vi "run order display.vi"() -> ()   [LabVIEW 2016]
doc: "Displays Run Order for editting and monitoring"
uses:
  datarunorder.ctl
  <vilib>/Utility/miscctls.llb/LVRowAndColumnTypeDef.ctl
  <vilib>/addons/database/Connection.llb/DB Tools Open Connec (String).vi
  <vilib>/addons/database/Connection.llb/Conn Execute.vi
  <vilib>/addons/database/Recordset.llb/Rec Fetch Recordset Data (R).vi
  <vilib>/addons/database/Recordset.llb/Rec Destroy - Connection.vi
  <vilib>/addons/database/NI_Database_API.lvlib
panel:
  in  "Tab Control":enum32{"Main", "Arrays and data"}(tab)
  in  "stop":bool
  out "Time Remaining Property error":errorcluster
  out "Estimated Time Remaining(min)":sgl format="%#.1f"
  out "sequences remaining":u8(slide) scale=0.0..80.0
  in  "run order display":T1
  in  "edit run list":i32(listbox)
  in  "Total time for each sequence(min)":dbl
  out "Estimated Wheel Finish time and Date":timestamp format="%<%I:%M %p\n%x>T"
  out "Total number of sequence":i32
  out "Sequence remaining":i32
  out "Add Holder error":errorcluster
  out "empty?":bool
  in  "add holder":T2
  in  "update wheel numbers":bool
  out "position change":u32[][](array[colorbox])
  out "position":u32
  out "subarray 2":string[](array[string])
  in  "create wheel file":bool
  out "Add Holder error 2":errorcluster
  out "Array":i32[](array[numeric])
  out "Group run list":string[][](array[string])
  out "Data":T3(array[cluster])
  out "subarray":string[](array[string])
  out "outofrange":bool
  out "cathode data":string[](array[string])
  out "recordset data":variant[][](array[variant])
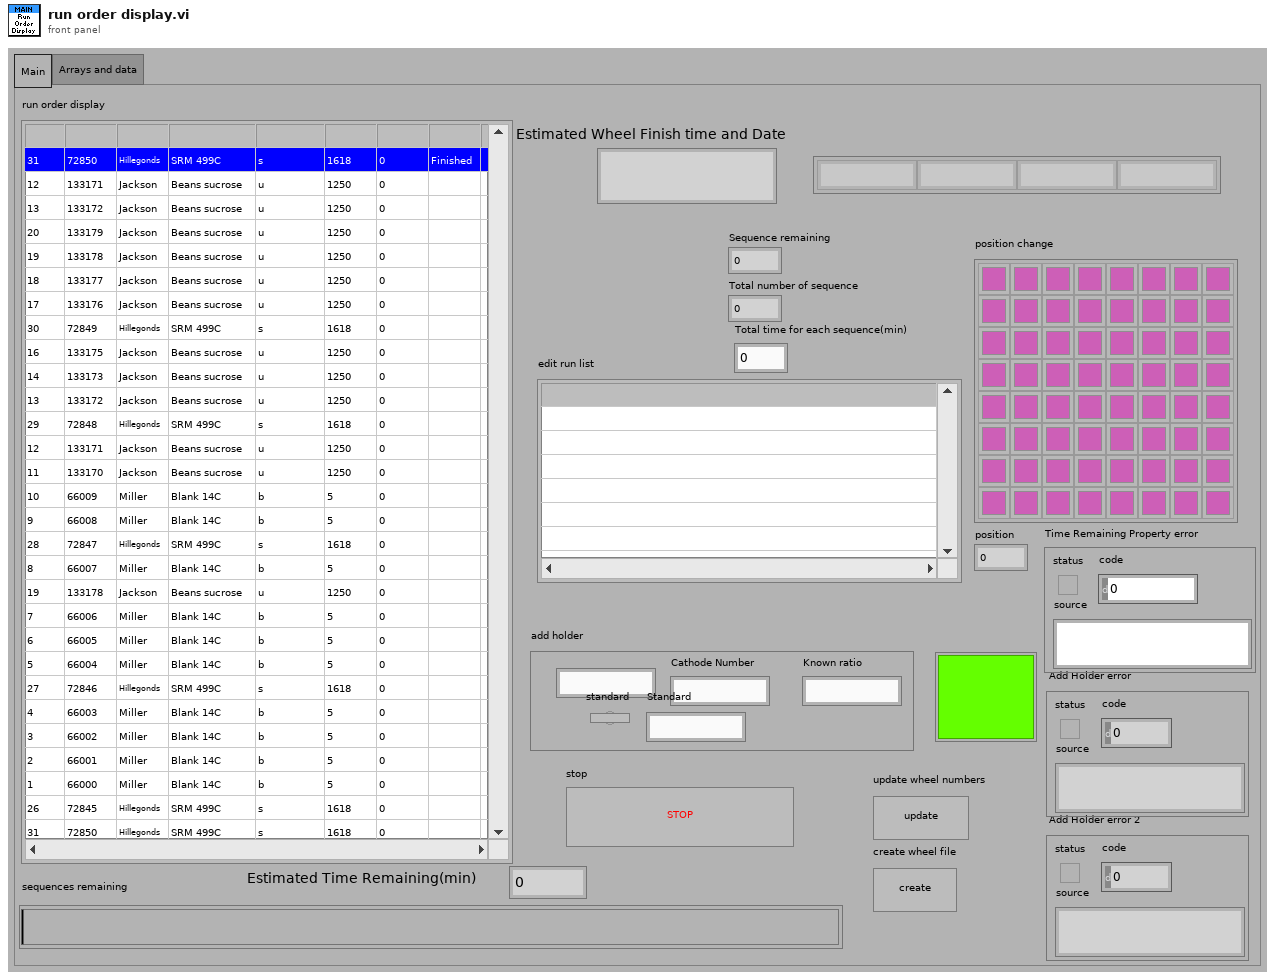
[diagram p1: front panel]
types:
  T1 = typedef "datarunorder.ctl" = i32
  T2 = cluster{"position":string, "Cathode Number":string, "standard":bool, "Known ratio":string, "Standard":string}
  T3 = cluster{"data name":string, "drag data":variant}[]
  T4 = typedef "LVRowAndColumnTypeDef.ctl" = cluster{"Row":i32, "Column":i32}
  T5 = typedef "LVPoint32TypeDef.ctl" = cluster{"Horizontal":i32, "Vertical":i32}
  T6 = typedef "NI_Database_API.lvlib/Conn ObjectReference.ctl" = refnum<k1>
  T7 = typedef "NI_Database_API.lvlib/Rec ObjectReference.ctl" = refnum<k1>
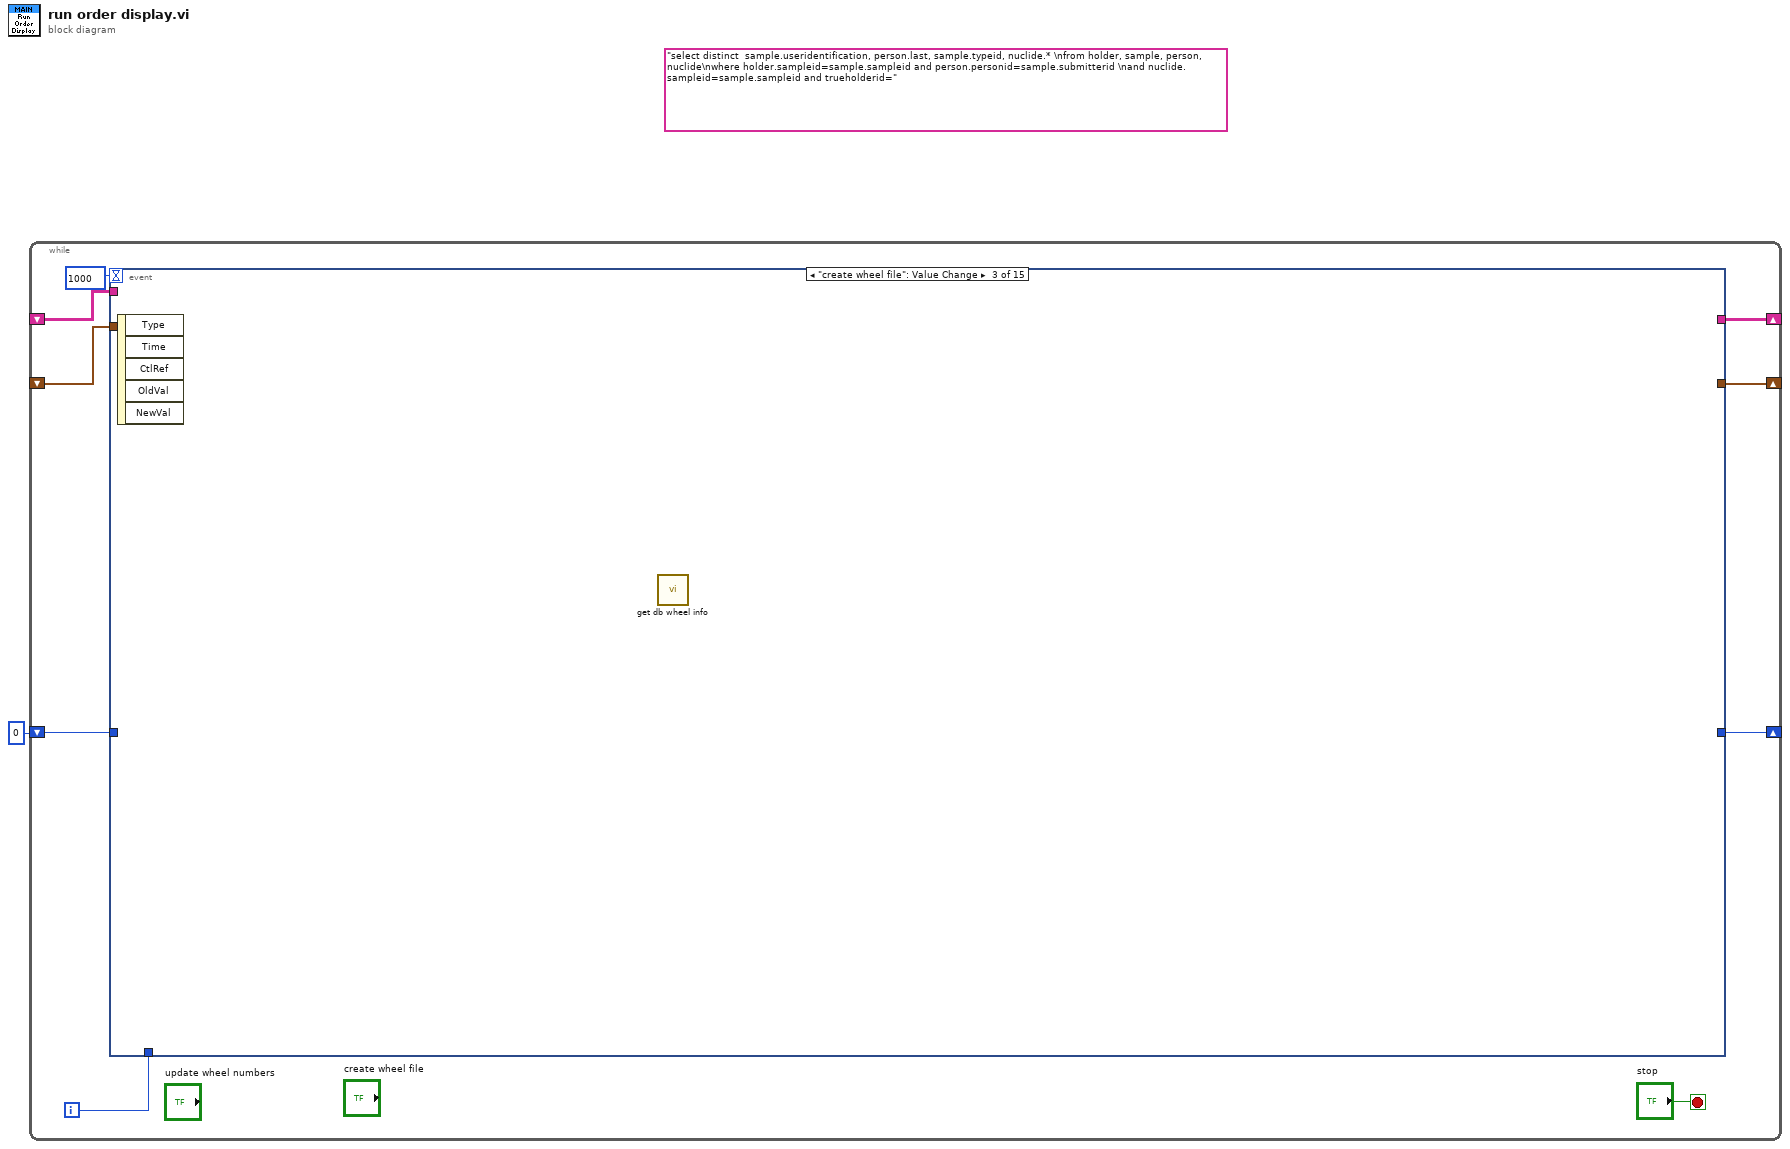
[diagram p0: block diagram]
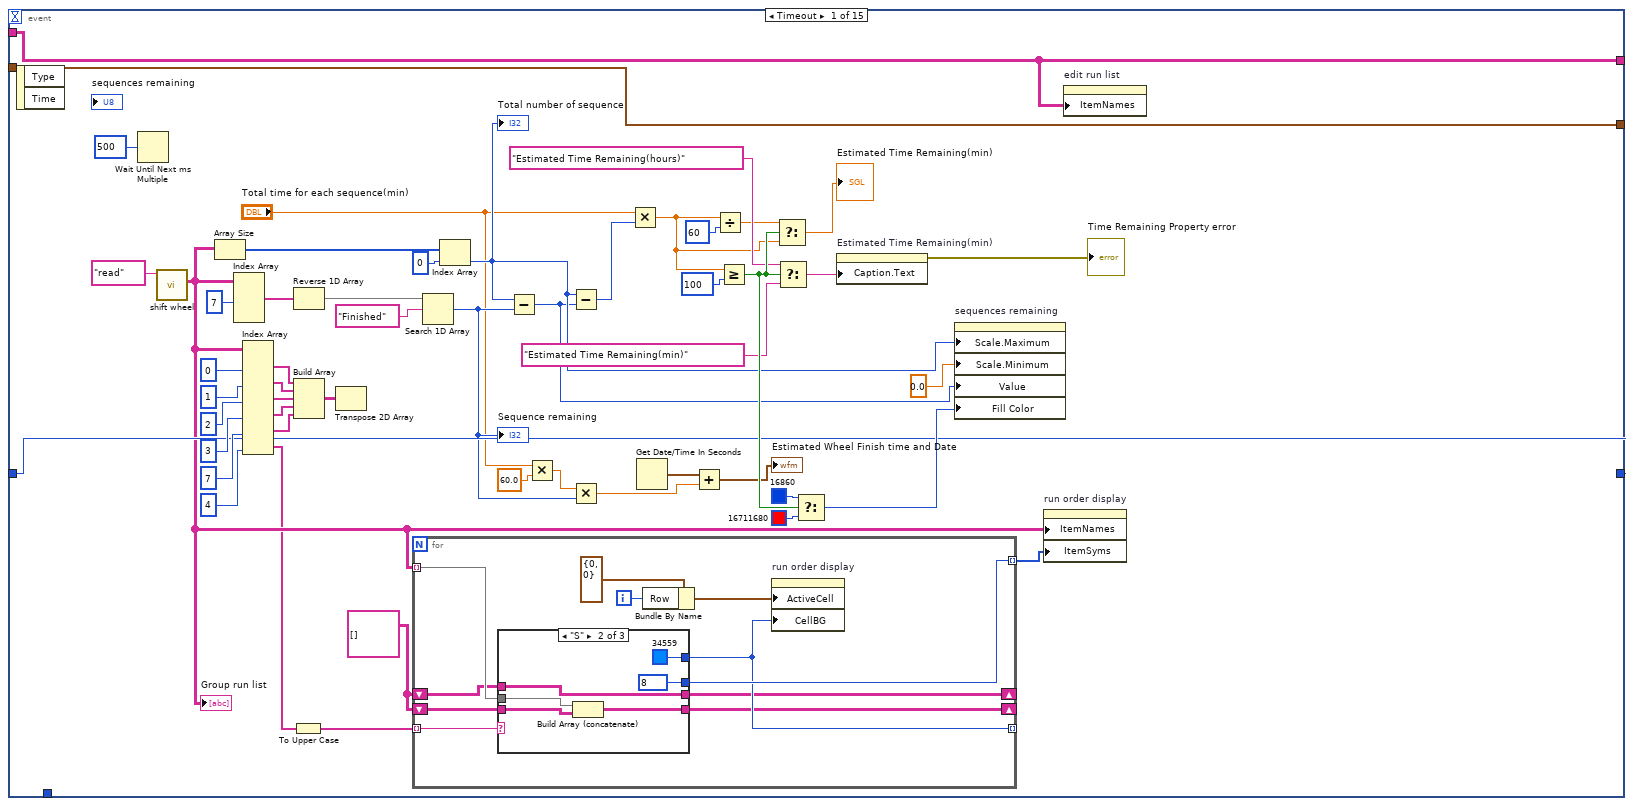
[diagram p2: hidden frame]
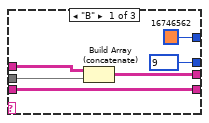
[diagram p3: hidden frame]
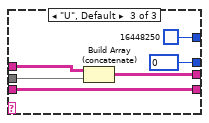
[diagram p4: hidden frame]
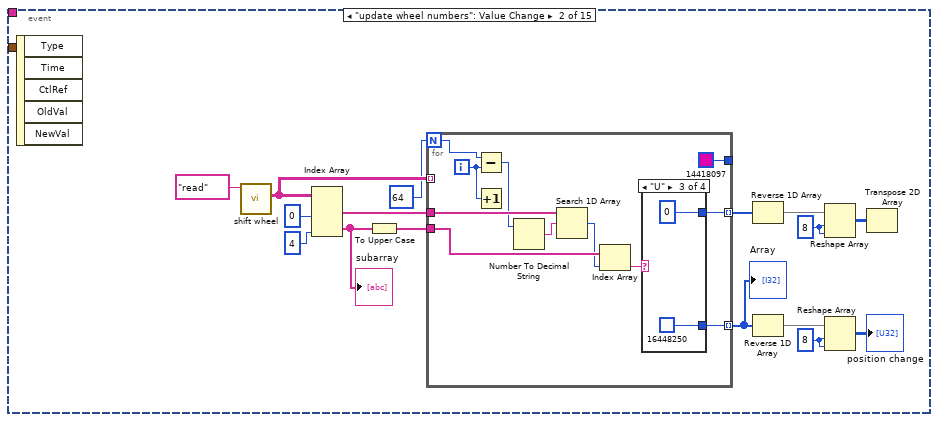
[diagram p5: hidden frame]
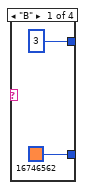
[diagram p6: hidden frame]
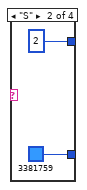
[diagram p7: hidden frame]
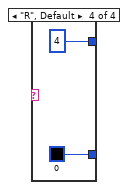
[diagram p8: hidden frame]
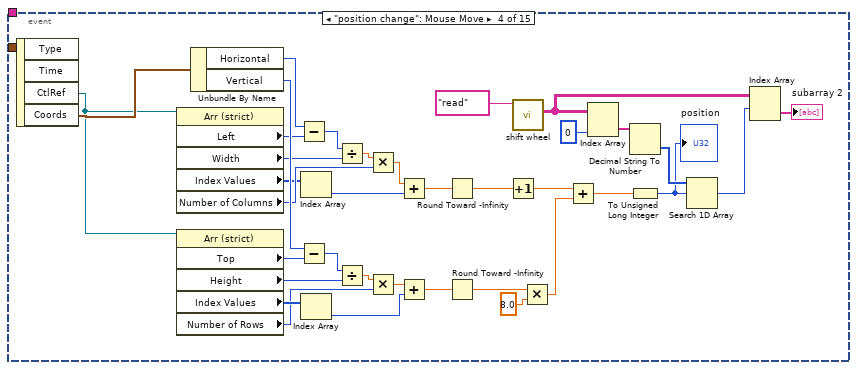
[diagram p9: hidden frame]
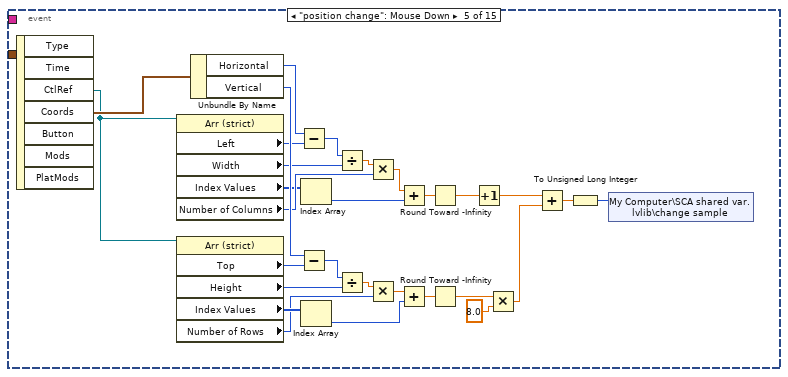
[diagram p10: hidden frame]
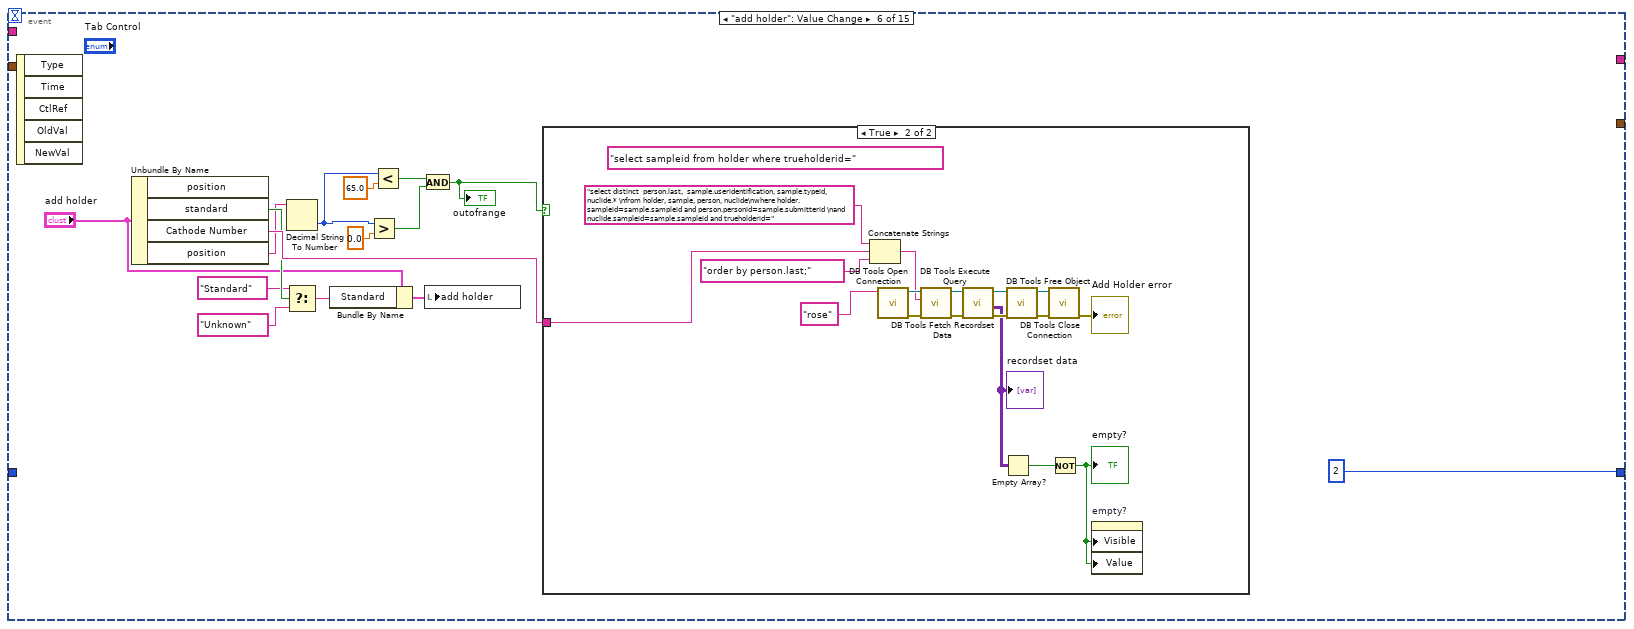
[diagram p11: hidden frame]
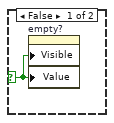
[diagram p12: hidden frame]
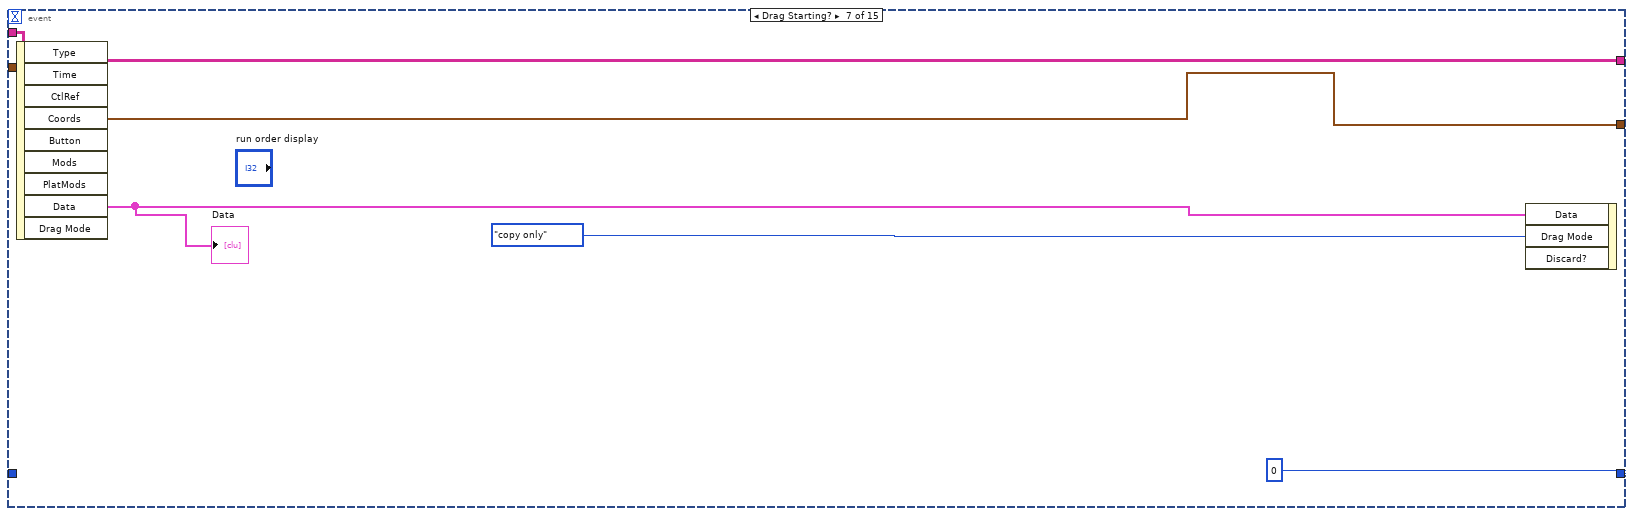
[diagram p13: hidden frame]
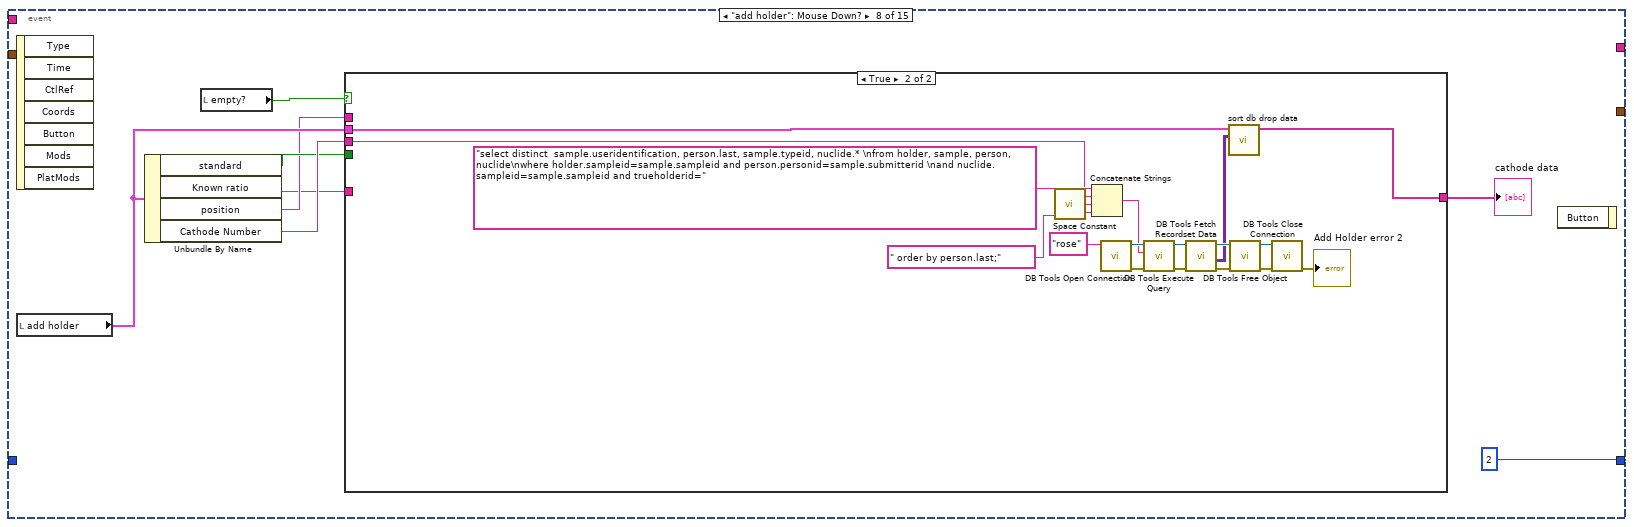
[diagram p14: hidden frame]
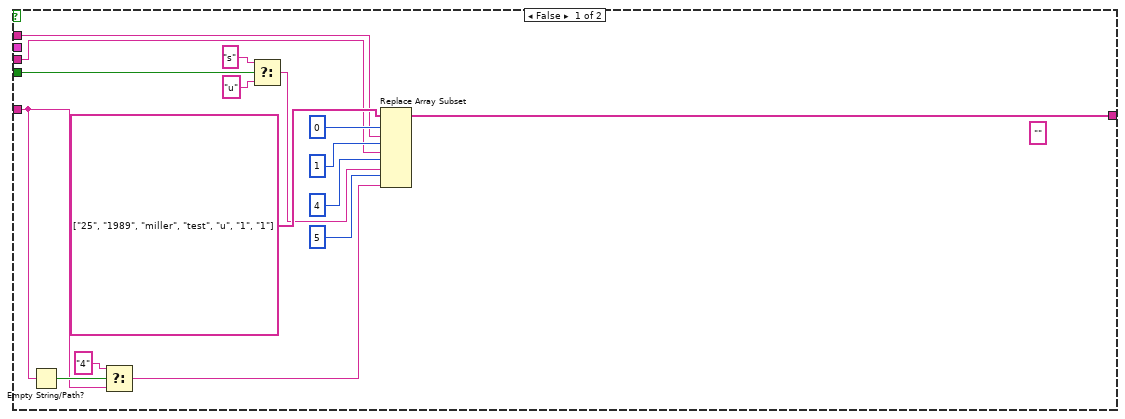
[diagram p15: hidden frame]
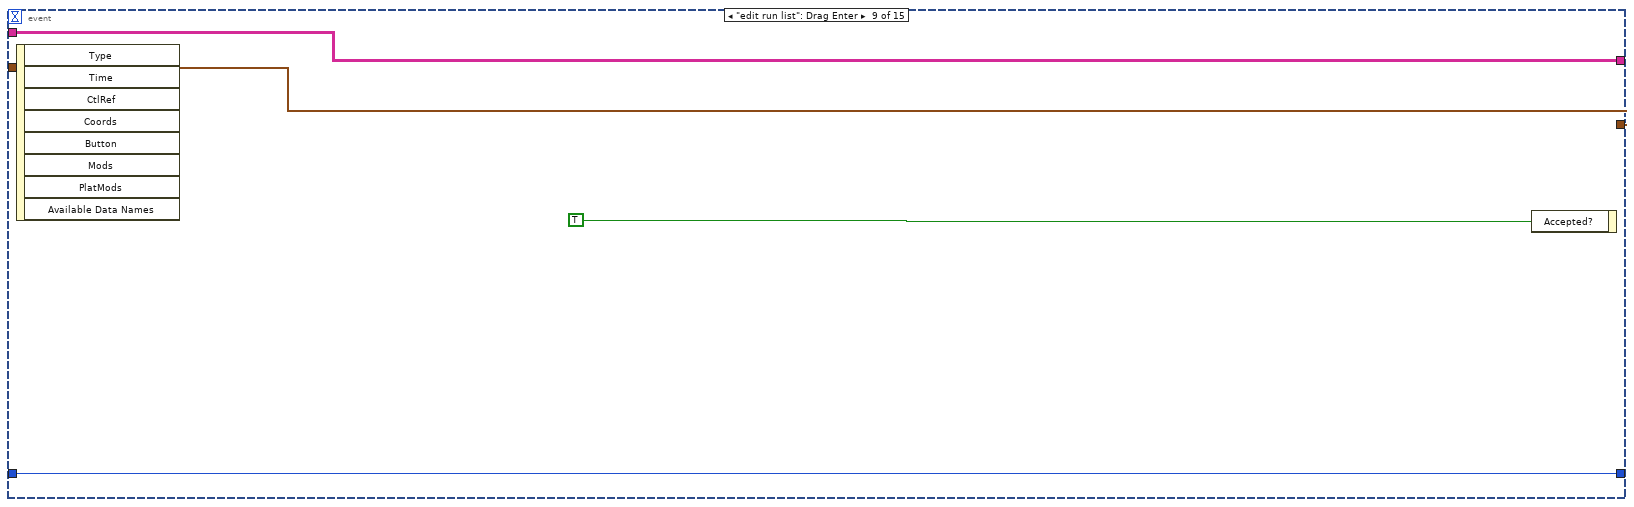
[diagram p16: hidden frame]
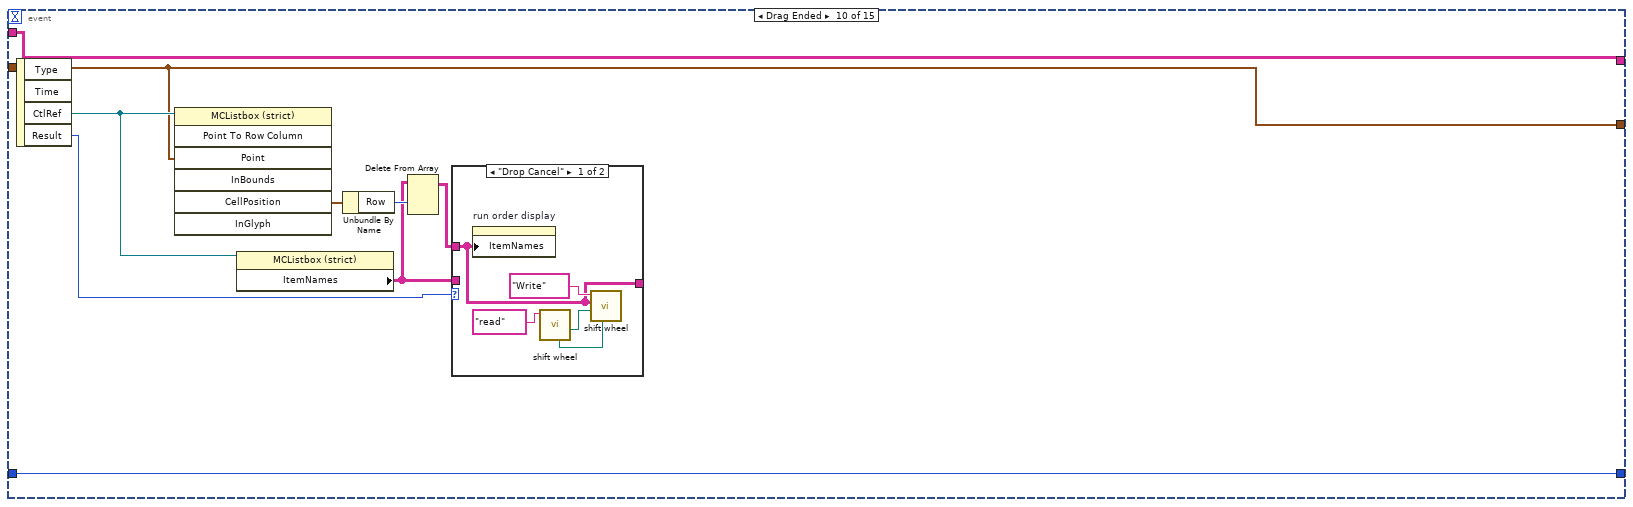
[diagram p17: hidden frame]
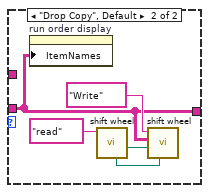
[diagram p18: hidden frame]
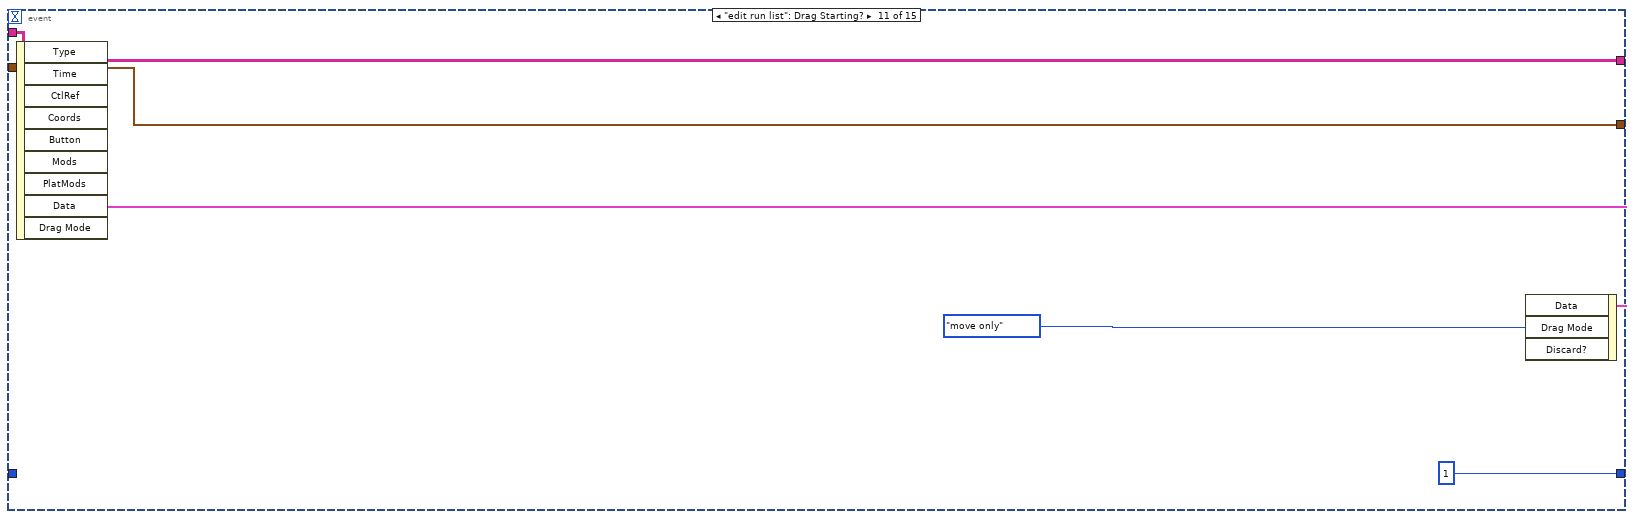
[diagram p19: hidden frame]
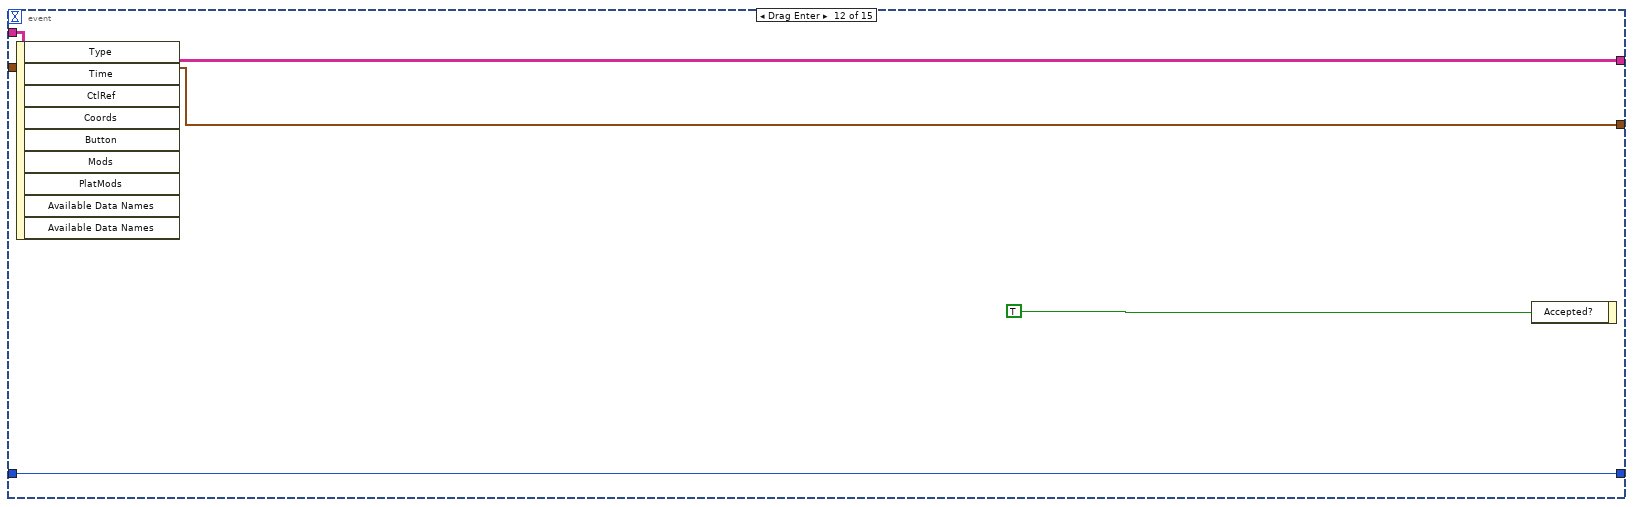
[diagram p20: hidden frame]
diagram:
  (unwired) "select distinct  sample.useridentification, person.last, sample.typeid, nuclide.* \nfrom holder, sample, person, nuclide\nwhere holder.sampleid=sample.sampleid and person.personid=sample.submitterid \nand nuclide.sampleid=sample.sampleid and trueholderid="
  n1 = while {
    shift-right: [w8] -> _
    shift-left: _ -> [w7]
    shift-right: [w6] -> _
    shift-left: _ -> [w5]
    shift-right: [w4] -> _
    shift-left: 0 -> [w3]
    i -> [w2]
    stop <- "stop" stop-if-true
    n2 = event shown="[2] \"create wheel file\": Value Change" {
      selector: _ -> [_ _ _ _ _ _ _ _ _ _ _ _ _ _ _]
      dyn-events: _ -> [_ _ _ _ _ _ _ _ _ _ _ _ _ _ _]
      timeout: 1000 -> [_ _ _ _ _ _ _ _ _ _ _ _ _ _ _]
      tunnel: w2 -> [_ _ _ _ _ _ _ _ _ _ _ _ _ _ _]
      tunnel: [w18 _ _ _ _ _ w228 _ w274 w277 w297 w302 _ _ w411] -> w8
      tunnel: w7 -> [w18 _ _ _ _ _ w228 _ w274 w277 w297 w302 w306 w356 w410]
      tunnel: [w62 _ _ _ _ _ w226 _ w273 w283 w296 w301 w315 w361 w406] -> w6
      tunnel: w5 -> [w62 _ _ _ _ _ _ _ w273 w283 w296 w301 w315 w361 w406]
      tunnel: [w26 _ _ _ _ 2 0 2 w272 w276 1 w300 0 0 w405] -> w4
      tunnel: w3 -> [w26 _ _ _ _ _ _ _ w272 w276 _ w300 w308 w359 w405]
      event Timeout {
        w15 = string[][] []
        n3 = event-data() -> ()  [unwired: 1 in, 2 out]
        n4 = Wait Until Next ms Multiple(millisecond multiple=u32 500) -> ()  [unwired: 1 out]
        n5 = call "shift wheel.vi"("read write"="read") -> ("Group run list"=w16:string[][])  [unwired: 8 in, 2 out]
        "Group run list" <- w16
        n6 = Array Size(array=w16) -> (size(s)=w28:i32[])
        n7 = Index Array(array=w16, index (col) #1=7 ("disabled index (col)")) -> (element #1=w31:string[])  [unwired: 3 in, 1 out]
        n8 = Index Array(array=w16, index (col) #1=0 ("disabled index (col)"), index (col) #2=1 ("index (col)"), index (col) #3=2 ("index (col)"), index (col) #4=3 ("index (col)"), index (col) #5=7 ("index (col)"), index (col) #6=4 ("index (col)")) -> (element #1=w56:string[], element #2=w57:string[], element #3=w58:string[], element #4=w59:string[], element #5=w60:string[], element #6=w13:string[])  [unwired: 6 in]
        n9 = To Upper Case(1:w13) -> (0:w12:string[])
        n10 = Reverse 1D Array(array=w31) -> (reversed array=w32:string[])
        n11 = Build Array(w56, w57, w58, w59, w60) -> (w61:string[][])
        n12 = Transpose 2D Array(2D array=w61) -> ()  [unwired: 1 out]
        n13 = for {
          tunnel: w12 -> [w73] mode=indexing
          tunnel: [w72] -> w14 mode=indexing
          tunnel: [w69] -> _ mode=indexing
          tunnel: w16 -> [w67] mode=indexing
          shift-right: [w66] -> _
          shift-left: w15 -> [w65]
          shift-right: [w64] -> _
          shift-left: w15 -> [w63]
          i -> [w68]
          n14 = case shown="\"S\"" w73 {
            tunnel: [9 8 0] -> w72
            tunnel: [u32 16746562 u32 34559 u32 16448250] -> w69
            tunnel: w67 -> [w74 w82 w88]
            tunnel: [w77 w83 w87] -> w66
            tunnel: w65 -> [w75 w83 w89]
            tunnel: [w76 w81 w86] -> w64
            tunnel: w63 -> [w76 w80 w86]
            frame "B" {
              n15 = Build Array (concatenate)(w75, w74) -> (w77:string[][])
            }
            frame "S" {
              n16 = Build Array (concatenate)(w82, w80) -> (w81:string[][])
            }
            frame "U", Default {
              n17 = Build Array (concatenate)(w89, w88) -> (w87:string[][])
            }
          }
          n18 = Bundle By Name(cluster=T4 {"Row"=0, "Column"=0} ("Active Cell:Active Cell"), "Row"=w68) -> (w71:T4)
          n19 = property on="run order display" class="MCListbox (strict)"("ActiveCell"=w71, "CellBG"=w69) -> ()  [unwired: 2 in, 2 out]
        }
        n20 = Search 1D Array(1D array=w32, element="Finished") -> (index of element=w20:i32)  [unwired: 1 in]
        "Sequence remaining" <- w20
        n21 = Index Array(array=w28, index=0) -> (element=w36:i32)
        "Total number of sequence" <- w36
        n22 = Subtract(x=w36, y=w20) -> (x-y=w24:i32)
        n23 = Multiply(x="Total time for each sequence(min)", y=60.0) -> (x*y=w22:dbl)
        n24 = Subtract(x=w36, y=w24) -> (x-y=w37:i32)
        n25 = Multiply(x=w22, y=w20) -> (x*y=w21:dbl)
        n26 = Multiply(x="Total time for each sequence(min)", y=w37) -> (x*y=w39:dbl)
        n27 = Get Date/Time In Seconds() -> (seconds since 1Jan1904=w25:timestamp)
        n28 = Add(x=w25, y=w21) -> (x+y=→"Estimated Wheel Finish time and Date":timestamp)
        n29 = Divide(x=w39, y=60) -> (x/y=w41:dbl)
        n30 = Greater Or Equal?(x=w39, y=100) -> (x >= y?=w49:bool)
        n31 = Select(t=w41, s=w49, f=w39) -> (s? t:f=→"Estimated Time Remaining(min)":dbl)
        n32 = Select(t="Estimated Time Remaining(hours)" ("Label.Text"), s=w49, f="Estimated Time Remaining(min)" ("Label.Text")) -> (s? t:f=w46:string)
        n33 = Select(t=u32 16860 ("Color Box"), s=w49, f=u32 16711680 ("Color Box 2")) -> (s? t:f=w50:u32)
        n34 = property on="Estimated Time Remaining(min)" class="DigNum (strict)"("Caption.Text"=w46) -> (error out=→"Time Remaining Property error":errorcluster)  [unwired: 2 in, 1 out]
        n35 = property on="sequences remaining" class="Slide (strict)"("Scale.Maximum"=w36, "Scale.Minimum"=0.0 ("Scale.Range:Minimum"), "Value"=w24, "Fill Color"=w50) -> ()  [unwired: 2 in, 2 out]
        n36 = property on="run order display" class="MCListbox (strict)"("ItemNames"=w16, "ItemSyms"=w14) -> ()  [unwired: 2 in, 2 out]
        n37 = property on="edit run list" class="MCListbox (strict)"("ItemNames"=w18) -> ()  [unwired: 2 in, 2 out]
      }
      event "update wheel numbers": Value Change {
        w96 = 8 ("dimension size")
        w99 = 8 ("dimension size")
        n38 = event-data() -> ()  [unwired: 1 in, 5 out]
        n39 = call "shift wheel.vi"("read write"="read") -> ("Group run list"=w106:string[][])  [unwired: 8 in, 2 out]
        n40 = Index Array(array=w106, index (col) #1=0 ("disabled index (col)"), index (col) #2=4 ("index (col)")) -> (element #1=w103:string[], element #2=w101:string[])  [unwired: 2 in]
        "subarray" <- w101
        n41 = To Upper Case(1:w101) -> (0:w100:string[])
        n42 = for {
          N: 64 -> [w112]
          tunnel: w106 -> [_] mode=indexing
          tunnel: w103 -> [w118]
          tunnel: w100 -> [w116]
          tunnel: [w113] -> w98 mode=indexing
          tunnel: [u32 14418097 ("Color Box")] -> _
          tunnel: [w108] -> w95 mode=indexing
          i -> [w111]
          n43 = Subtract(x=w112, y=w111) -> (x-y=w110:i32)
          n44 = Increment(x=w111) -> ()  [unwired: 1 out]
          n45 = Number To Decimal String(number=w110) -> (decimal integer string=w117:string)  [unwired: 1 in]
          n46 = Search 1D Array(1D array=w118, element=w117) -> (index of element=w115:i32)  [unwired: 1 in]
          n47 = Index Array(array=w116, index=w115) -> (element=w114:string)
          n48 = case shown="\"U\"" w114 {
            tunnel: [u32 16746562 ("Color Box") u32 3381759 ("Color Box") u32 16448250 ("Color Box") u32 0 ("Color Box")] -> w113
            tunnel: [3 ("x") 2 ("x") 0 ("x") 4 ("x")] -> w108
            frame "B" {
            }
            frame "S" {
            }
            frame "U" {
            }
            frame "R", Default {
            }
          }
        }
        "Array" <- w98
        n49 = Reverse 1D Array(array=w95) -> (reversed array=w94:i32[])
        n50 = Reverse 1D Array(array=w98) -> (reversed array=w97:u32[])
        n51 = Reshape Array(w94, w96, w96) -> (w93:i32[][])
        n52 = Reshape Array(w97, w99, w99) -> (→"position change":u32[][])
        n53 = Transpose 2D Array(2D array=w93) -> ()  [unwired: 1 out]
      }
      event "create wheel file": Value Change {
        n54 = event-data() -> ()  [unwired: 1 in, 5 out]
        n55 = call "get db wheel info.vi"() -> ()  [unwired: 1 in]
      }
      event "position change": Mouse Move {
        n56 = event-data() -> ("CtlRef"=w151:refnum<vi>, "Coords"=w161:T5)  [unwired: 1 in, 2 out]
        n57 = property class="Arr (strict)"(reference=w151) -> ("Left"=w145:i32, "Width"=w143:u32, "Index Values"=w141:u32[], "Number of Columns"=w142:u32)  [unwired: 1 in, 2 out]
        n58 = property class="Arr (strict)"(reference=w151) -> ("Top"=w159:i32, "Height"=w157:u32, "Index Values"=w156:u32[], "Number of Rows"=w155:u32)  [unwired: 1 in, 2 out]
        n59 = Unbundle By Name(w161) -> ("Horizontal"=w144:i32, "Vertical"=w160:i32)
        n60 = Subtract(x=w144, y=w145) -> (x-y=w147:i32)
        n61 = Subtract(x=w160, y=w159) -> (x-y=w158:i32)
        n62 = Index Array(array=w141) -> (element=w149:u32)  [unwired: 1 in]
        n63 = Index Array(array=w156) -> (element=w153:u32)  [unwired: 1 in]
        n64 = Divide(x=w147, y=w143) -> (x/y=w148:dbl)
        n65 = Divide(x=w158, y=w157) -> (x/y=w154:dbl)
        n66 = Multiply(x=w148, y=w142) -> (x*y=w150:dbl)
        n67 = Multiply(x=w154, y=w155) -> (x*y=w152:dbl)
        n68 = Add(x=w150, y=w149) -> (x+y=w146:dbl)
        n69 = Add(x=w152, y=w153) -> (x+y=w162:dbl)
        n70 = Round Toward -Infinity(1:w146) -> (0:w137:dbl)
        n71 = Round Toward -Infinity(1:w162) -> (0:w140:dbl)
        n72 = Increment(x=w137) -> (x+1=w136:dbl)
        n73 = call "shift wheel.vi"("read write"="read") -> ("Group run list"=w130:string[][])  [unwired: 8 in, 2 out]
        n74 = Multiply(x=w140, y=8.0) -> (x*y=w138:dbl)
        n75 = Add(x=w136, y=w138) -> (x+y=w133:dbl)
        n76 = Index Array(array=w130, index (col)=0 ("disabled index (col)")) -> (element=w134:string[])  [unwired: 1 in]
        n77 = Decimal String To Number(string=w134) -> (number=w132:i32[])  [unwired: 2 in, 1 out]
        n78 = To Unsigned Long Integer(number=w133) -> (unsigned 32bit integer=w131:u32)
        "position" <- w131
        n79 = Search 1D Array(1D array=w132, element=w131) -> (index of element=w129:i32)  [unwired: 1 in]
        n80 = Index Array(array=w130, index (row)=w129) -> (element=→"subarray 2":string[])  [unwired: 1 in]
      }
      event "position change": Mouse Down {
        n81 = event-data() -> ("CtlRef"=w180:refnum<vi>, "Coords"=w190:T5)  [unwired: 1 in, 5 out]
        n82 = property class="Arr (strict)"(reference=w180) -> ("Left"=w174:i32, "Width"=w172:u32, "Index Values"=w170:u32[], "Number of Columns"=w171:u32)  [unwired: 1 in, 2 out]
        n83 = property class="Arr (strict)"(reference=w180) -> ("Top"=w188:i32, "Height"=w186:u32, "Index Values"=w185:u32[], "Number of Rows"=w184:u32)  [unwired: 1 in, 2 out]
        n84 = Unbundle By Name(w190) -> ("Horizontal"=w173:i32, "Vertical"=w189:i32)
        n85 = Subtract(x=w173, y=w174) -> (x-y=w176:i32)
        n86 = Subtract(x=w189, y=w188) -> (x-y=w187:i32)
        n87 = Index Array(array=w170) -> (element=w178:u32)  [unwired: 1 in]
        n88 = Index Array(array=w185) -> (element=w182:u32)  [unwired: 1 in]
        n89 = Divide(x=w176, y=w172) -> (x/y=w177:dbl)
        n90 = Divide(x=w187, y=w186) -> (x/y=w183:dbl)
        n91 = Multiply(x=w177, y=w171) -> (x*y=w179:dbl)
        n92 = Multiply(x=w183, y=w184) -> (x*y=w181:dbl)
        n93 = Add(x=w179, y=w178) -> (x+y=w175:dbl)
        n94 = Add(x=w181, y=w182) -> (x+y=w191:dbl)
        n95 = Round Toward -Infinity(1:w175) -> (0:w166:dbl)
        n96 = Round Toward -Infinity(1:w191) -> (0:w169:dbl)
        n97 = Increment(x=w166) -> (x+1=w165:dbl)
        n98 = Multiply(x=w169, y=8.0) -> (x*y=w167:dbl)
        n99 = Add(x=w165, y=w167) -> (x+y=w164:dbl)
        n100 = To Unsigned Long Integer(number=w164) -> (unsigned 32bit integer=w163:u32)
        n101 = shared-variable "My Computer\\SCA shared var.lvlib\\change sample"(w163) -> ()  [unwired: 1 in, 1 out]
      }
      event "add holder": Value Change {
        n102 = event-data() -> ()  [unwired: 1 in, 5 out]
        n103 = Unbundle By Name("add holder") -> ("standard"=w202:bool, "Cathode Number"=w203:string, "position"=w196:string)  [unwired: 1 out]
        n104 = Decimal String To Number(string=w196) -> (number=w195:i32)  [unwired: 2 in, 1 out]
        n105 = Select(t="Standard" ("decimal integer string"), s=w202, f="Unknown" ("decimal integer string")) -> (s? t:f=w199:string)
        n106 = Bundle By Name(cluster="add holder", "Standard"=w199) -> (w198:T2)
        n107 = Greater?(x=w195, y=0.0) -> (0:w206:bool)
        n108 = Less?(x=w195, y=65.0) -> (x < y?=w205:bool)
        n109 = And(x=w205, y=w206) -> (x .and. y?=w204:bool)
        "outofrange" <- w204
        n110 = local write "add holder"(w198) -> ()
        n111 = case shown="True" w204 {
          selector: w204 -> [w207 _]
          tunnel: w203 -> [_ w211]
          frame False {
            n112 = property on="empty?" class="Bool (strict)"("Visible"=w207, "Value"=w207) -> ()  [unwired: 2 in, 2 out]
          }
          frame True {
            (unwired) "select sampleid from holder where trueholderid=" ("SQL query")
            n113 = Concatenate Strings("select distinct  person.last,  sample.useridentification, sample.typeid, nuclide.* \nfrom holder, sample, person, nuclide\nwhere holder.sampleid=sample.sampleid and person.personid=sample.submitterid \nand nuclide.sampleid=sample.sampleid and trueholderid=", w211, "order by person.last;" ("string")) -> (w219:string)
            n114 = call-poly <vilib>:"DB Tools Open Connection.vi"("connection information"="rose" ("decimal integer string")) -> ("error out"=w224:errorcluster, "connection reference"=w223:T6)  [unwired: 7 in]
            n115 = call-poly <vilib>:"DB Tools Execute Query.vi"("error in (no error)"=w224, "SQL query"=w219, "connection reference"=w223) -> ("error out"=w222:errorcluster, "recordset reference"=w221:T7)  [unwired: 5 in]
            n116 = call-poly <vilib>:"DB Tools Fetch Recordset Data.vi"("error in (no error)"=w222, "recordset reference"=w221) -> ("error out"=w218:errorcluster, "recordset data"=w213:variant[][], "recordset reference out"=w217:T7)  [unwired: 3 in]
            "recordset data" <- w213
            n117 = Empty Array?(array=w213) -> (empty?=w209:bool)
            n118 = call-poly <vilib>:"DB Tools Free Object.vi"("error in (no error)"=w218, "recordset reference"=w217) -> ("error out"=w216:errorcluster, "connection reference"=w215:T6)  [unwired: 8 in]
            n119 = call <vilib>:"DB Tools Close Connection.vi"("error in (no error)"=w216, "connection reference"=w215) -> ("error out"=→"Add Holder error":errorcluster)  [unwired: 5 in]
            n120 = Not(x=w209) -> (.not. x?=w208:bool)
            "empty?" <- w208
            n121 = property on="empty?" class="Bool (strict)"("Visible"=w208, "Value"=w208) -> ()  [unwired: 2 in, 2 out]
          }
        }
      }
      event Drag Starting? {
        n122 = event-data() -> ("Coords"=w226:T5, "Data"=w229:T3)  [unwired: 1 in, 7 out]
        "Data" <- w229
        n123 = event-data("Data"=w229, "Drag Mode"=enum32{"copy or move", "copy only", "move only"}."copy only") -> ()  [unwired: 2 in, 1 out]
      }
      event "add holder": Mouse Down? {
        n124 = event-data() -> ()  [unwired: 1 in, 7 out]
        n125 = local read "add holder"() -> (w235:T2)
        n126 = Unbundle By Name(w235) -> ("standard"=w233:bool, "Known ratio"=w231:string, "position"=w232:string, "Cathode Number"=w236:string)
        n127 = local read "empty?"() -> (w237:bool)
        n128 = case shown="True" w237 {
          tunnel: w236 -> [w246 w259]
          tunnel: w235 -> [_ w255]
          tunnel: [w238 w254] -> w230
          tunnel: w233 -> [w252 _]
          tunnel: w232 -> [w247 _]
          tunnel: w231 -> [w241 _]
          frame False {
            (unwired) "" ("new element/subarray")
            n129 = Empty String/Path?(string/path=w241) -> (empty?=w242:bool)
            n130 = Select(t="4" ("new element/subarray"), s=w242, f=w241) -> (s? t:f=w239:string)
            n131 = Select(t="s", s=w252, f="u") -> (s? t:f=w244:string)
            n132 = Replace Array Subset(array=string[] ["25", "1989", "miller", "test", "u", "1", "1"] ("cathode data"), new element #1=w247, index #1=0 ("index"), new element #2=w246, index #2=1 ("index"), new element #3=w244, index #3=4 ("index"), new element #4=w239, index #4=5 ("index")) -> (w238:string[])
          }
          frame True {
            n133 = call <vilib>:"Space Constant.vi"() -> ("String"=w257:string)
            n134 = Concatenate Strings("select distinct  sample.useridentification, person.last, sample.typeid, nuclide.* \nfrom holder, sample, person, nuclide\nwhere holder.sampleid=sample.sampleid and person.personid=sample.submitterid \nand nuclide.sampleid=sample.sampleid and trueholderid=", w259, w257, " order by person.last;" ("string")) -> (w263:string)
            n135 = call-poly <vilib>:"DB Tools Open Connection.vi"("connection information"="rose" ("decimal integer string")) -> ("error out"=w270:errorcluster, "connection reference"=w269:T6)  [unwired: 7 in]
            n136 = call-poly <vilib>:"DB Tools Execute Query.vi"("error in (no error)"=w270, "SQL query"=w263, "connection reference"=w269) -> ("error out"=w268:errorcluster, "recordset reference"=w267:T7)  [unwired: 5 in]
            n137 = call-poly <vilib>:"DB Tools Fetch Recordset Data.vi"("error in (no error)"=w268, "recordset reference"=w267) -> ("error out"=w262:errorcluster, "recordset data"=w256:variant[][], "recordset reference out"=w266:T7)  [unwired: 3 in]
            n138 = call "sort db drop data.vi"("recordset data"=w256, "add holder"=w255) -> ("cathode data"=w254:string[])  [unwired: 8 in, 1 out]
            n139 = call-poly <vilib>:"DB Tools Free Object.vi"("error in (no error)"=w262, "recordset reference"=w266) -> ("error out"=w261:errorcluster, "connection reference"=w265:T6)  [unwired: 8 in]
            n140 = call <vilib>:"DB Tools Close Connection.vi"("error in (no error)"=w261, "connection reference"=w265) -> ("error out"=→"Add Holder error 2":errorcluster)  [unwired: 5 in]
          }
        }
        "cathode data" <- w230
        n141 = event-data() -> ()  [unwired: 2 in, 1 out]
      }
      event "edit run list": Drag Enter {
        n142 = event-data() -> ()  [unwired: 1 in, 8 out]
        n143 = event-data("Accepted?"=TRUE) -> ()  [unwired: 1 in, 1 out]
      }
      event Drag Ended {
        n144 = event-data() -> ("CtlRef"=w284:refnum<vi>, "Result"=w279:enum16{"Drop Cancel", "Drop Move", "Drop Copy"})  [unwired: 1 in, 2 out]
        n145 = invoke class="MCListbox (strict)" method="Point To Row Column"(reference=w284, "Point"=w283) -> ("CellPosition"=w282:T4)  [unwired: 5 in, 6 out]
        n146 = property class="MCListbox (strict)"(reference=w284) -> ("ItemNames"=w278:string[][])  [unwired: 1 in, 2 out]
        n147 = Unbundle By Name(w282) -> ("Row"=w281:i32)
        n148 = Delete From Array(array=w278, index (row)=w281) -> (array with subset deleted=w280:string[][])  [unwired: 2 in, 1 out]
        n149 = case shown="\"Drop Cancel\"" w279 {
          tunnel: w280 -> [w285 _]
          tunnel: [w285 w290] -> _
          tunnel: w278 -> [_ w290]
          frame "Drop Cancel" {
            n150 = property on="run order display" class="MCListbox (strict)"("ItemNames"=w285) -> ()  [unwired: 2 in, 2 out]
            n151 = call "shift wheel.vi"("read write"="read") -> ("cycle results name out"=w288:path, "seq results name out"=w289:path)  [unwired: 8 in, 1 out]
            n152 = call "shift wheel.vi"("seq results name in"=w289, "cycle results name in"=w288, "Group run list write"=w285, "read write"="Write") -> ()  [unwired: 5 in, 3 out]
          }
          frame "Drop Copy", Default {
            n153 = property on="run order display" class="MCListbox (strict)"("ItemNames"=w290) -> ()  [unwired: 2 in, 2 out]
            n154 = call "shift wheel.vi"("read write"="read") -> ("cycle results name out"=w293:path, "seq results name out"=w294:path)  [unwired: 8 in, 1 out]
            n155 = call "shift wheel.vi"("seq results name in"=w294, "cycle results name in"=w293, "Group run list write"=w290, "read write"="Write") -> ()  [unwired: 5 in, 3 out]
          }
        }
      }
      event "edit run list": Drag Starting? {
        n156 = event-data() -> ("Data"=w299:T3)  [unwired: 1 in, 8 out]
        n157 = event-data("Data"=w299, "Drag Mode"=enum32{"copy or move", "copy only", "move only"}."move only") -> ()  [unwired: 2 in, 1 out]
      }
      event Drag Enter {
        n158 = event-data() -> ()  [unwired: 1 in, 9 out]
        n159 = event-data("Accepted?"=TRUE) -> ()  [unwired: 1 in, 1 out]
      }
      event Drop {
        (unwired) 0 ("index")
        n160 = event-data() -> ("CtlRef"=w325:refnum<vi>, "Coords"=w324:T5, "Available Data Names"=w310:string[])  [unwired: 1 in, 7 out]
        n161 = case shown="0, Default" w308 {
          tunnel: [w327 w352 w353] -> w307
          tunnel: w306 -> [_ w352 _]
          frame 0, Default {
            (unwired) "" ("delimiter (Tab)")
            n162 = local read "Data"() -> (w351:T3)
            n163 = Index Array(array=w351, index=1) -> (element=w349:cluster{"data name":string, "drag data":variant})
            n164 = Unbundle By Name(w349) -> ("drag data"=w332:variant)
            n165 = Variant To Flattened String(Variant=w332) -> (data string=w346:string)  [unwired: 1 out]
            n166 = String Subset(string=w346, offset (0)=8, length (rest)=2 ("length (rest)")) -> (substring=w343:string)
            n167 = call <vilib>:"Trim Whitespace.vi"("string"=w343) -> ("trimmed string"=w333:string)  [unwired: 1 in]
            n168 = String To Byte Array(string=w333) -> (unsigned byte array=w340:u8[])
            n169 = Search 1D Array(1D array=w340, element=u8 0) -> (index of element=w339:i32)  [unwired: 1 in]
            n170 = Array Subset(array=w340, length=w339) -> (w338:u8[])  [unwired: 1 in]
            n171 = Equal?(x=w339, y=-1) -> (x = y?=w341:bool)
            n172 = property on="run order display" class="MCListbox (strict)"() -> ("ItemNames"=w335:string[][])  [unwired: 2 in, 2 out]
            n173 = Select(t=w340, s=w341, f=w338) -> (s? t:f=w337:u8[])
            n174 = Byte Array To String(unsigned byte array=w337) -> (string=w336:string)
            n175 = Index Array(array=w335, index (col)=0 ("disabled index (col)")) -> (element=w344:string[])  [unwired: 1 in]
            n176 = Search 1D Array(1D array=w344, element=w336) -> (index of element=w334:i32)  [unwired: 1 in]
            n177 = Index Array(array=w335, index (row)=w334) -> (element=w331:string[])  [unwired: 1 in]
            n178 = Array Subset(array=w331, length=7) -> (w328:string[])  [unwired: 1 in]
            n179 = Build Array(w328) -> (w327:string[][])
          }
          frame 1 {
            n180 = property on="edit run list" class="MCListbox (strict)" props=["ItemNames"]() -> ()  [unwired: 2 in, 3 out]
          }
          frame 2 {
            n181 = property on="edit run list" class="MCListbox (strict)" props=["ItemNames"]() -> ()  [unwired: 2 in, 3 out]
            n182 = local read "cathode data"() -> (w354:string[])
            n183 = Build Array(w354) -> (w353:string[][])
          }
        }
        n184 = Index Array(array=w310, index=1) -> ()  [unwired: 1 out]
        n185 = property on="run order display" class="MCListbox (strict)"() -> ("ItemNames"=w319:string[][])  [unwired: 2 in, 2 out]
        n186 = invoke class="MCListbox (strict)" method="Point To Row Column"(reference=w325, "Point"=w324) -> ("CellPosition"=w323:T4)  [unwired: 5 in, 6 out]
        n187 = Unbundle By Name(w323) -> ("Row"=w318:i32)
        n188 = Array Subset(array=w319, index (row)=0 ("index"), length (row)=w318) -> (w317:string[][])  [unwired: 2 in]
        n189 = Array Size(array=w319) -> (size(s)=w322:i32[])
        n190 = Array Subset(array=w319, index (row)=w318) -> (w316:string[][])  [unwired: 3 in]
        n191 = Index Array(array=w322, index=0) -> ()  [unwired: 1 out]
        n192 = Build Array (concatenate)(w317, w307, w316) -> (w304:string[][])
        n193 = property on="run order display" class="MCListbox (strict)"("ItemNames"=w304) -> ()  [unwired: 2 in, 2 out]
        n194 = call "shift wheel.vi"("read write"="read") -> ("cycle results name out"=w313:path, "seq results name out"=w312:path)  [unwired: 8 in, 1 out]
        n195 = call "shift wheel.vi"("seq results name in"=w312, "cycle results name in"=w313, "Group run list write"=w304, "read write"="Write") -> ()  [unwired: 5 in, 3 out]
        n196 = event-data("Accepted?"=TRUE) -> ()  [unwired: 1 in, 1 out]
      }
      event Mouse Up {
        n197 = event-data() -> ("CtlRef"=w371:refnum<vi>, "Coords"=w370:T5)  [unwired: 1 in, 5 out]
        n198 = case shown="0, Default" w359 {
          tunnel: [w377 w402 w403] -> w358
          tunnel: w356 -> [_ w402 _]
          frame 0, Default {
            (unwired) "" ("delimiter (Tab)")
            n199 = local read "Data"() -> (w401:T3)
            n200 = Index Array(array=w401, index=1) -> (element=w399:cluster{"data name":string, "drag data":variant})
            n201 = Unbundle By Name(w399) -> ("drag data"=w382:variant)
            n202 = Variant To Flattened String(Variant=w382) -> (data string=w396:string)  [unwired: 1 out]
            n203 = String Subset(string=w396, offset (0)=8, length (rest)=2 ("length (rest)")) -> (substring=w393:string)
            n204 = call <vilib>:"Trim Whitespace.vi"("string"=w393) -> ("trimmed string"=w383:string)  [unwired: 1 in]
            n205 = String To Byte Array(string=w383) -> (unsigned byte array=w390:u8[])
            n206 = Search 1D Array(1D array=w390, element=u8 0) -> (index of element=w389:i32)  [unwired: 1 in]
            n207 = property on="run order display" class="MCListbox (strict)"() -> ("ItemNames"=w385:string[][])  [unwired: 2 in, 2 out]
            n208 = Array Subset(array=w390, length=w389) -> (w388:u8[])  [unwired: 1 in]
            n209 = Equal?(x=w389, y=-1) -> (x = y?=w391:bool)
            n210 = Select(t=w390, s=w391, f=w388) -> (s? t:f=w387:u8[])
            n211 = Byte Array To String(unsigned byte array=w387) -> (string=w386:string)
            n212 = Index Array(array=w385, index (col)=0 ("disabled index (col)")) -> (element=w394:string[])  [unwired: 1 in]
            n213 = Search 1D Array(1D array=w394, element=w386) -> (index of element=w384:i32)  [unwired: 1 in]
            n214 = Index Array(array=w385, index (row)=w384) -> (element=w381:string[])  [unwired: 1 in]
            n215 = Array Subset(array=w381, length=7) -> (w378:string[])  [unwired: 1 in]
            n216 = Build Array(w378) -> (w377:string[][])
          }
          frame 1 {
            n217 = property on="edit run list" class="MCListbox (strict)" props=["ItemNames"]() -> ()  [unwired: 2 in, 3 out]
          }
          frame 2 {
            n218 = property on="edit run list" class="MCListbox (strict)" props=["ItemNames"]() -> ()  [unwired: 2 in, 3 out]
            n219 = local read "cathode data"() -> (w404:string[])
            n220 = Build Array(w404) -> (w403:string[][])
          }
        }
        n221 = invoke class="MCListbox (strict)" method="Point To Row Column"(reference=w371, "Point"=w370) -> ("CellPosition"=w369:T4)  [unwired: 5 in, 6 out]
        n222 = property on="run order display" class="MCListbox (strict)"() -> ("ItemNames"=w365:string[][])  [unwired: 2 in, 2 out]
        n223 = Unbundle By Name(w369) -> ("Row"=w364:i32)
        n224 = Array Size(array=w365) -> (size(s)=w368:i32[])
        n225 = Array Subset(array=w365, index (row)=w364) -> (w362:string[][])  [unwired: 3 in]
        n226 = Array Subset(array=w365, index (row)=0 ("index"), length (row)=w364) -> (w363:string[][])  [unwired: 2 in]
        n227 = local read "outofrange"() -> (w355:bool)
        n228 = Index Array(array=w368, index=0) -> ()  [unwired: 1 out]
        n229 = Build Array (concatenate)(w363, w358, w362) -> (w357:string[][])
        n230 = property on="run order display" class="MCListbox (strict)"("ItemNames"=w357) -> ()  [unwired: 2 in, 2 out]
        n231 = case shown="True" w355 {
          tunnel: w357 -> [_ w372]
          frame False {
          }
          frame True {
            (unwired) TRUE ("Accepted?")
            n232 = call "shift wheel.vi"("read write"="read") -> ("cycle results name out"=w374:path, "seq results name out"=w373:path)  [unwired: 8 in, 1 out]
            n233 = call "shift wheel.vi"("seq results name in"=w373, "cycle results name in"=w374, "Group run list write"=w372, "read write"="Write") -> ()  [unwired: 5 in, 3 out]
          }
        }
      }
      event "edit run list": Drop {
        n234 = event-data() -> ()  [unwired: 1 in, 9 out]
        n235 = local read "Data"() -> (w433:T3)
        n236 = Index Array(array=w433, index=1) -> (element=w431:cluster{"data name":string, "drag data":variant})
        n237 = Unbundle By Name(w431) -> ("drag data"=w412:variant)
        n238 = Variant To Flattened String(Variant=w412) -> (data string=w428:string)  [unwired: 1 out]
        n239 = String Subset(string=w428, offset (0)=8, length (rest)=2 ("length (rest)")) -> (substring=w425:string)
        n240 = call <vilib>:"Trim Whitespace.vi"("string"=w425) -> ("trimmed string"=w413:string)  [unwired: 1 in]
        n241 = String To Byte Array(string=w413) -> (unsigned byte array=w421:u8[])
        n242 = Search 1D Array(1D array=w421, element=u8 0) -> (index of element=w420:i32)  [unwired: 1 in]
        n243 = property on="run order display" class="MCListbox (strict)"() -> ("ItemNames"=w415:string[][])  [unwired: 2 in, 2 out]
        n244 = Array Subset(array=w421, length=w420) -> (w419:u8[])  [unwired: 1 in]
        n245 = Equal?(x=w420, y=-1) -> (x = y?=w423:bool)
        n246 = Select(t=w421, s=w423, f=w419) -> (s? t:f=w418:u8[])
        n247 = Byte Array To String(unsigned byte array=w418) -> (string=w417:string)
        n248 = Index Array(array=w415, index (col)=0 ("disabled index (col)")) -> (element=w426:string[])  [unwired: 1 in]
        n249 = Search 1D Array(1D array=w426, element=w417) -> (index of element=w414:i32)  [unwired: 1 in]
        n250 = Index Array(array=w415, index (row)=w414) -> (element=w409:string[])  [unwired: 1 in]
        n251 = Array Subset(array=w409, length=7) -> (w407:string[])  [unwired: 1 in]
        n252 = Build Array (concatenate)(w410, w407) -> (w411:string[][])
        n253 = event-data("Accepted?"=TRUE) -> ()  [unwired: 1 in, 1 out]
      }
    }
  }
